vi "Intake Controller.vi"(8 "error in":errorcluster) -> ()   [LabVIEW 2015]
doc: "This VI executes continuously carrying out the current operation and responding to updates or new operations. It will often contain the timing or control code that is difficult to place directly in TeleOp. This VI generally opens all sensors and motors and isolates the rest of the robot code from knowing how the operations are carried out."
uses:
  Intake Setpoints.ctl
  Intake Operations.ctl
  <vilib>/Rock Robotics/WPI/CAN/TalonSRX/WPI_CANTalonSRX_APIControlMode.ctl
  <vilib>/Rock Robotics/WPI/SafetyOutput/WPI_SafetyOutputConfigMenu.ctl
  <vilib>/Rock Robotics/SystemInterfaces/DIO/FPGA_DIOChannel.ctl
  Support Code/OnButton/OnButtonSingle.vi
  Intake Published Globals.vi
  <vilib>/Rock Robotics/WPI/MotorControl/WPI_MotorControlOpenCANTalonSRX.vi
  <vilib>/Rock Robotics/Network Tables/NT Write Boolean.vi
panel:
  out "Current\nCmd":string
  # "Tip: It may be helpful to observe inputs and sensor values.\nYou may also want to display tuning or debugging controls."
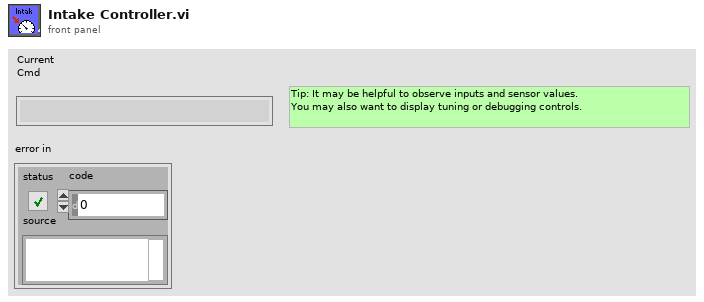
[diagram p1: front panel]
types:
  T1 = typedef "Intake Setpoints.ctl" = cluster{"Operation":T2, "Setpoint":dbl, "Duration":dbl}
  T2 = typedef "Intake Operations.ctl" = enum16{"Reserve", "Read Current", "Immediate", "Idle", "Eject", "Intake", "Queue to Shooter", "Load to Shooter"}
  T3 = typedef "FPGA_DIOChannel.ctl" = enum8{"DIO 0", "DIO 1", "DIO 2", "DIO 3", "DIO 4", "DIO 5", "DIO 6", "DIO 7", "DIO 8", "DIO 9", "DIO MXP 0", "DIO MXP 1", "DIO MXP 2", "DIO MXP 3", "DIO MXP 4", "DIO MXP 5", "DIO MXP 6", "DIO MXP 7", "DIO MXP 8", "DIO MXP 9", "DIO MXP 10", "DIO MXP 11", "DIO MXP 12", "DIO MXP 13", "DIO MXP 14", "DIO MXP 15", "Invalid"}
  T4 = typedef "WPI_SafetyOutputConfigMenu.ctl" = enum16{"Enable", "Disable"}
  T5 = typedef "WPI_CANTalonSRX_APIControlMode.ctl" = enum8{"Percent VBus", "Speed", "Position", "Slave", "Unchanged / Invalid", "Voltage Compensation", "Current", "Motion Profile"}
  T6 = typedef "WPI_DigitalInputDevRef.ctl" = cluster{"DevStatus":errorcluster, "DIO Channel":T3}
  T7 = typedef "WPI_MotorControlDeviceRef.ctl" = cluster{"DeviceStatus":errorcluster, "Type":T8, "PWM":cluster{"PWM Channel":T9, "DeadBand":T10}, "CAN":cluster{"Device Number":u8, "Control Mode":T11, "Semaphore":T12, "Max Vout":dbl, "TalonSRX Control Mode":T5}, "Invert":bool}
  T8 = typedef "WPI_MotorControlType.ctl" = enum16{"PWM", "CAN", "CANTalonSRX"}
  T9 = typedef "FPGA_DIOPWMChannel.ctl" = enum8{"PWM 0", "PWM 1", "PWM 2", "PWM 3", "PWM 4", "PWM 5", "PWM 6", "PWM 7", "PWM 8", "PWM 9", "PWM MXP 0", "PWM MXP 1", "PWM MXP 2", "PWM MXP 3", "PWM MXP 4", "PWM MXP 5", "PWM MXP 6", "PWM MXP 7", "PWM MXP 8", "PWM MXP 9", "Invalid"}
  T10 = typedef "WPI_PWMDeadband.ctl" = cluster{"Name":string, "maxPositivePwm":i32, "minPositivePwm":i32, "centerPwm":i32, "maxNegativePwm":i32, "minNegativePwm":i32, "angularRange":u16}
  T11 = typedef "WPI_CANJaguar_ControlMode.ctl" = enum8{"Percent VBus", "Current", "Speed", "Position", "Voltage"}
  T12 = typedef "Semaphore RefNum" = refnum<k1>
  T13 = typedef "Command Status Info.ctl" = cluster{"Name":string, "Status":T14, "notifier out":T15}
  T14 = typedef "Completion Status.ctl" = enum16{"Successful", "Aborted", "Incomplete"}
  T15 = typedef "Completion Notifier.ctl" = refnum<notifier>
  T16 = cluster{"Default Command":T1, "Command Timing":cluster{"Start Time (ms)":u32, "Iterations":i32}, "Command Arguments":cluster{"Command Info":T13, "Description":string, "Default Command":T1, "notifier out":refnum<notifier>, "Subsystem Name":string}}
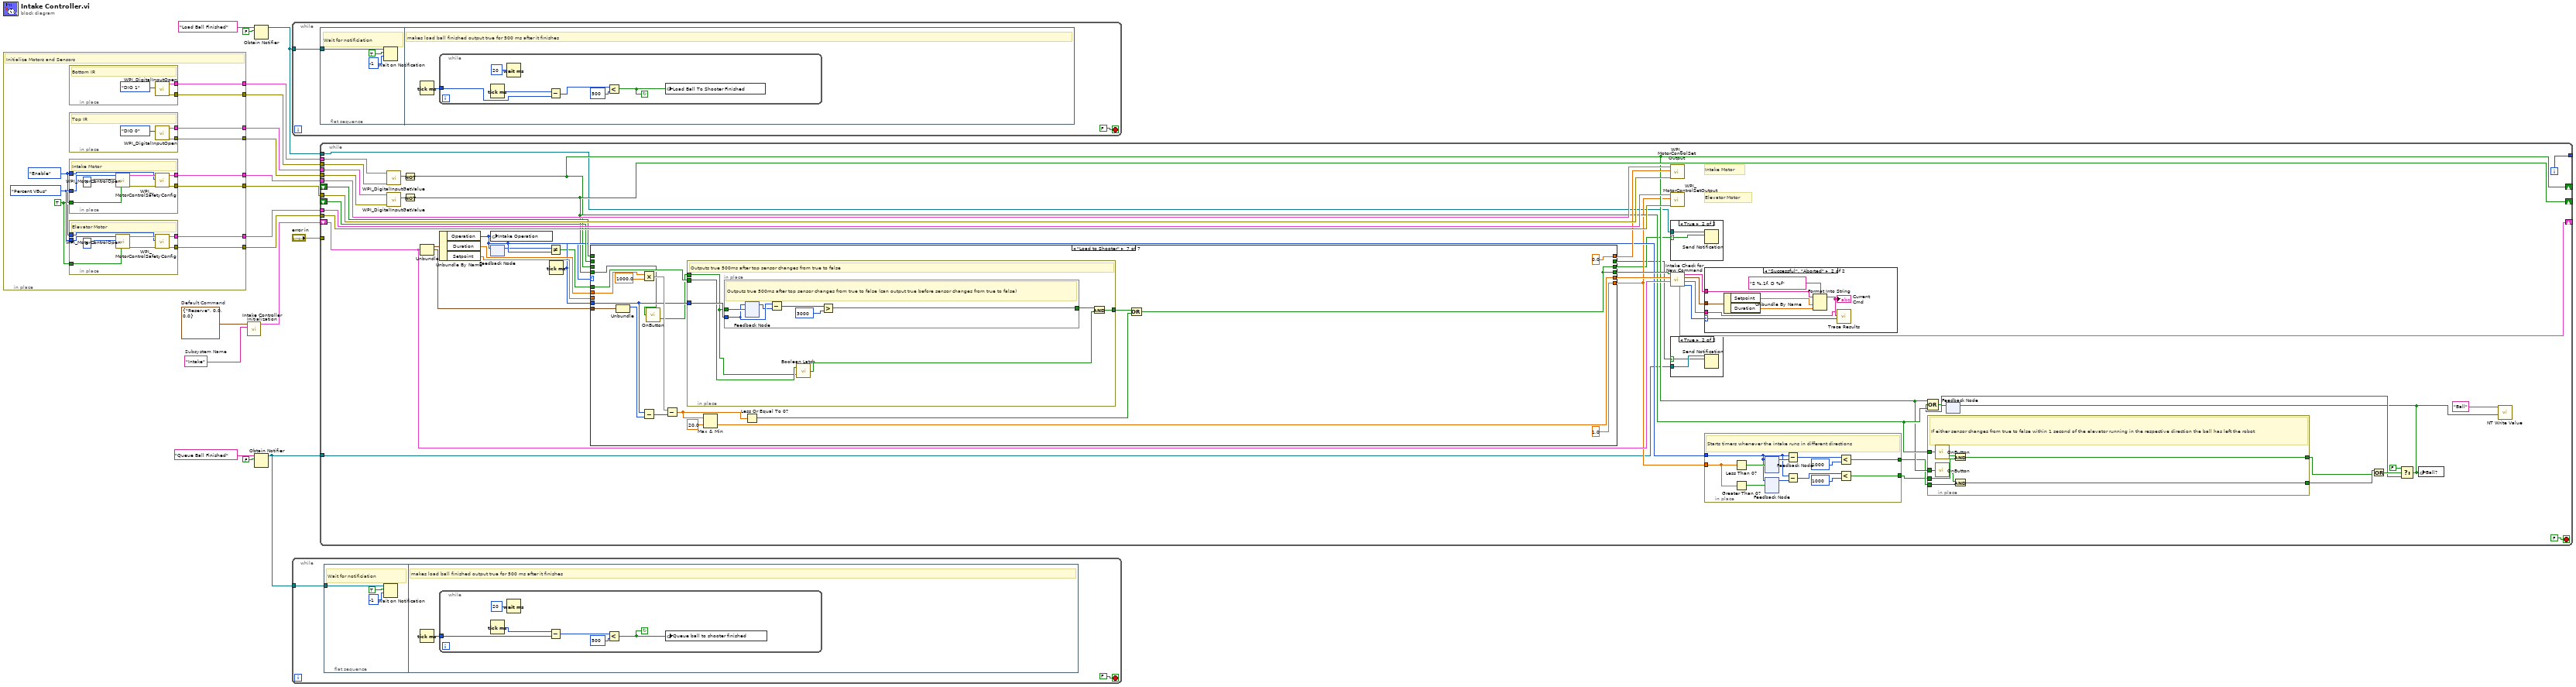
[diagram p0: block diagram]
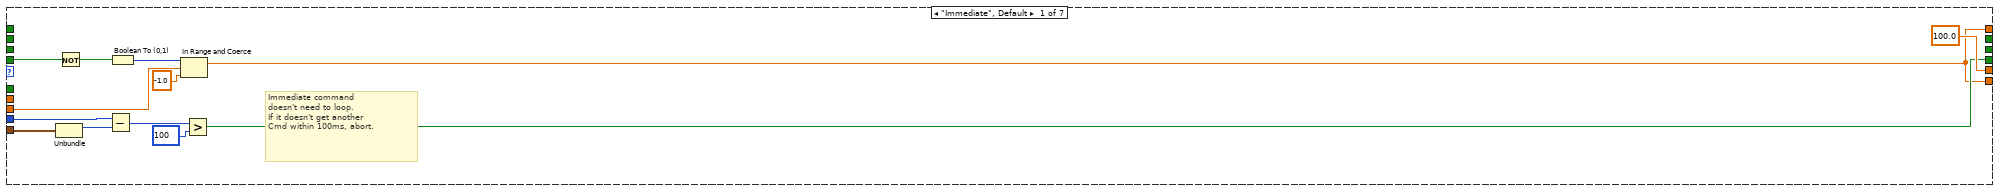
[diagram p5: hidden frame]
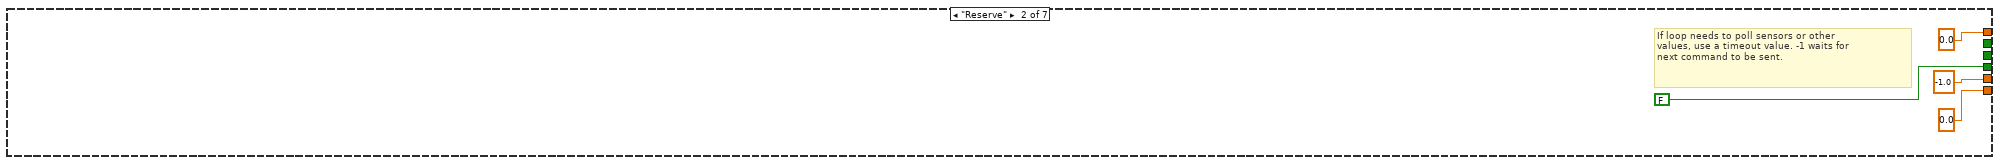
[diagram p6: hidden frame]
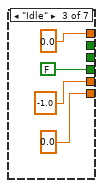
[diagram p7: hidden frame]
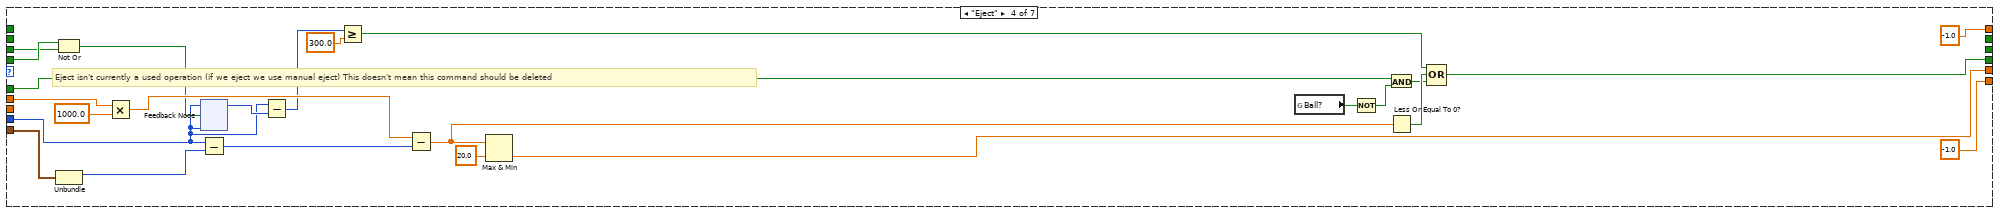
[diagram p8: hidden frame]
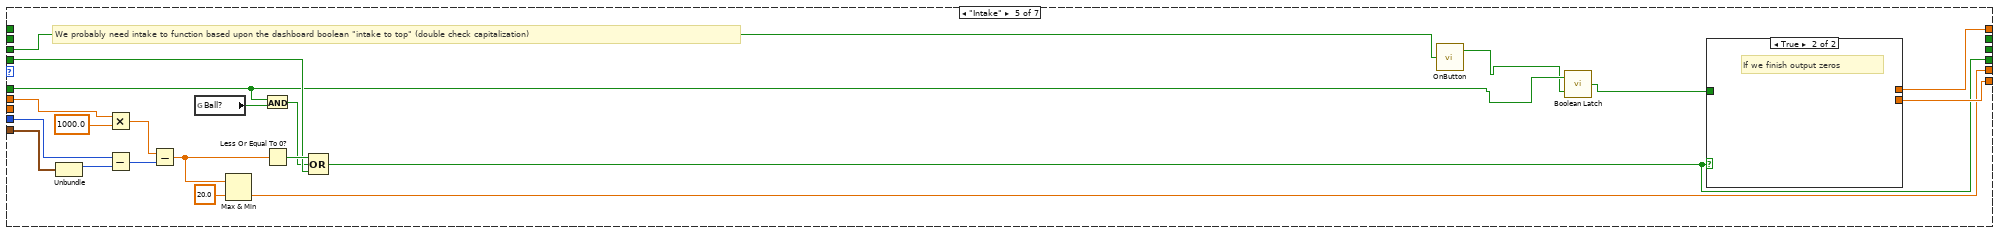
[diagram p9: hidden frame]
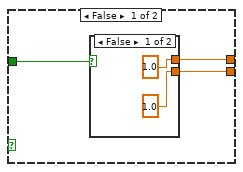
[diagram p10: hidden frame]
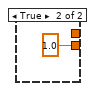
[diagram p11: hidden frame]
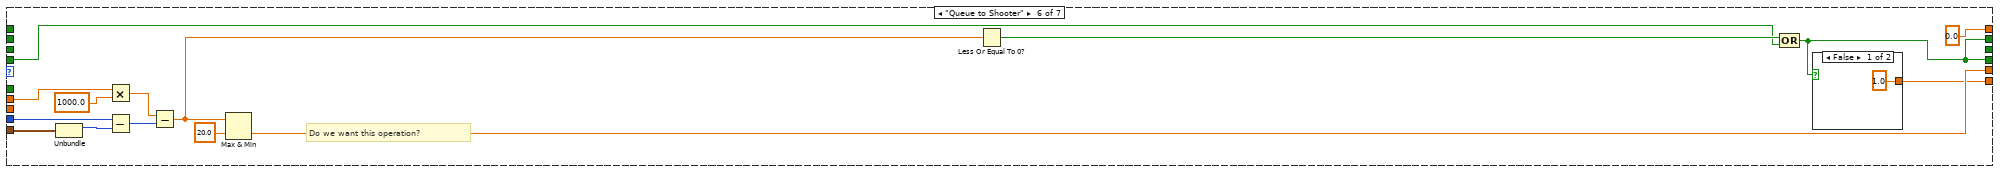
[diagram p12: hidden frame]
diagram:
  w15 = T1 {"Operation"=enum."Reserve", "Setpoint"=0.0, "Duration"=0.0}  # Default Command
  w16 = "Intake"  # Subsystem Name
  n1 = in-place {
    in-place-border: [w29] -> w14
    in-place-border: [w26] -> w13
    in-place-border: [w25] -> w12
    in-place-border: [w24] -> w11
    in-place-border: [w23] -> w10
    in-place-border: [w21] -> w9
    in-place-border: [w20] -> w8
    in-place-border: [w19] -> w7
    w22 = WPI_SafetyOutputConfigMenu."Enable" ("mode")
    w27 = TRUE ("Invert")
    w28 = WPI_CANTalonSRX_APIControlMode."Percent VBus" ("Control Mode")
    # "Initialize Motors and Sensors"
    n2 = in-place {
      in-place-border: [w35] -> w29
      in-place-border: [w34] -> w21
      # "Bottom IR"
      n3 = call <vilib>:"WPI_DigitalInputOpen.vi"("DIO Channel"=FPGA_DIOChannel."DIO 1") -> ("error out"=w34:errorcluster, "DigitalInputDevRef"=w35:T6)  [unwired: 9 in]
    }
    n4 = in-place {
      in-place-border: [w32] -> w20
      in-place-border: [w31] -> w19
      # "Top IR"
      n5 = call <vilib>:"WPI_DigitalInputOpen.vi"("DIO Channel"=FPGA_DIOChannel."DIO 0") -> ("error out"=w32:errorcluster, "DigitalInputDevRef"=w31:T6)  [unwired: 9 in]
    }
    n6 = in-place {
      in-place-border: w28 -> [w51]
      in-place-border: w27 -> [w50]
      in-place-border: [w48] -> w24
      in-place-border: [w46] -> w23
      in-place-border: w22 -> [w45]
      # "Intake Motor"
      n7 = call-poly <vilib>:"WPI_MotorControlOpen.vi"("Invert"=w50, "Device Number"=u8 7, "Control Mode"=w51) -> ("error out"=w49:errorcluster, "MotorControlDeviceRef"=w47:T7)  [unwired: 7 in]
      n8 = call <vilib>:"WPI_MotorControlSafetyConfig.vi"("error in (no error)"=w49, "mode"=w45, "MotorControlDevRef"=w47) -> ("error out"=w48:errorcluster, "MotorControlDevRef"=w46:T7)  [unwired: 7 in]
    }
    n9 = in-place {
      in-place-border: w28 -> [w43]
      in-place-border: w27 -> [w42]
      in-place-border: [w40] -> w26
      in-place-border: [w38] -> w25
      in-place-border: w22 -> [w37]
      # "Elevator Motor"
      n10 = call-poly <vilib>:"WPI_MotorControlOpen.vi"("Invert"=w42, "Device Number"=u8 8, "Control Mode"=w43) -> ("error out"=w39:errorcluster, "MotorControlDeviceRef"=w41:T7)  [unwired: 7 in]
      n11 = call <vilib>:"WPI_MotorControlSafetyConfig.vi"("error in (no error)"=w39, "mode"=w37, "MotorControlDevRef"=w41) -> ("error out"=w38:errorcluster, "MotorControlDevRef"=w40:T7)  [unwired: 7 in]
    }
  }
  n12 = call "Intake Controller Initialization.vi"("Subsystem Name"=w16, "Default Command"=w15) -> ("Command Info"=w17:T16)  [unwired: 9 in]
  n13 = Obtain Notifier(name (unnamed)="Load Ball Finished", notification data type=FALSE) -> (notifier out=w4:refnum<notifier>)  [unwired: 2 in, 2 out]
  n14 = Obtain Notifier(name (unnamed)="Queue Ball Finished", notification data type=FALSE) -> (notifier out=w1:refnum<notifier>)  [unwired: 2 in, 2 out]
  n15 = while {
    tunnel: w4 -> [w53]
    stop <- FALSE stop-if-true
    n16 = flat-sequence {
      tunnel: w53 -> [w56]
      frame #0 {
        # "Wait for notificiation"
        n17 = Wait on Notification(notifier=w56, ignore previous (F)=TRUE, timeout in ms (-1)=-1) -> ()  [unwired: 1 in, 4 out]
      }
      frame #1 {
        # "makes load ball finished output true for 500 ms after it finishes"
        n18 = Tick Count (ms)() -> (millisecond timer value=w57:u32)
        n19 = while {
          tunnel: w57 -> [w59]
          stop <- w63 continue-if-true
          n20 = Tick Count (ms)() -> (millisecond timer value=w58:u32)
          n21 = Wait (ms)(milliseconds to wait=20) -> ()  [unwired: 1 out]
          n22 = Subtract(x=w58, y=w59) -> (x-y=w61:u32)
          n23 = Less?(x=w61, y=u32 500) -> (x < y?=w63:bool)
          n24 = global write "Intake Published Globals.vi" "Load Ball To Shooter Finished"(w63) -> ()
        }
      }
    }
  }
  n25 = while {
    tunnel: w1 -> [w65]
    stop <- FALSE stop-if-true
    n26 = flat-sequence {
      tunnel: w65 -> [w68]
      frame #0 {
        # "Wait for notificiation"
        n27 = Wait on Notification(notifier=w68, ignore previous (F)=TRUE, timeout in ms (-1)=-1) -> ()  [unwired: 1 in, 4 out]
      }
      frame #1 {
        # "makes load ball finished output true for 500 ms after it finishes"
        n28 = Tick Count (ms)() -> (millisecond timer value=w69:u32)
        n29 = while {
          tunnel: w69 -> [w71]
          stop <- w75 continue-if-true
          n30 = Tick Count (ms)() -> (millisecond timer value=w70:u32)
          n31 = Wait (ms)(milliseconds to wait=20) -> ()  [unwired: 1 out]
          n32 = Subtract(x=w70, y=w71) -> (x-y=w73:u32)
          n33 = Less?(x=w73, y=u32 500) -> (x < y?=w75:bool)
          n34 = global write "Intake Published Globals.vi" "Queue ball to shooter finished"(w75) -> ()
        }
      }
    }
  }
  n35 = while {
    shift-right: [w116] -> _
    shift-left: w17 -> [w117]
    tunnel: [w122] -> _
    tunnel: "error in" -> [_]
    tunnel: w14 -> [w109]
    tunnel: w10 -> [w108]
    tunnel: w13 -> [w107]
    tunnel: w12 -> [w106]
    tunnel: w11 -> [w105]
    tunnel: w9 -> [w104]
    tunnel: w8 -> [w103]
    tunnel: w7 -> [w102]
    shift-right: [w95] -> _
    shift-left: _ -> [w99]
    shift-right: [w94] -> _
    shift-left: _ -> [w100]
    tunnel: w4 -> [w92]
    tunnel: w1 -> [w89]
    i -> [w122]
    stop <- FALSE stop-if-true
    # "Intake Motor"
    # "Elevator Motor"
    n36 = call <vilib>:"WPI_DigitalInputGetValue.vi"("error in (no error)"=w104, "DigitalInputDevRef"=w109) -> ("Value"=w76:bool)  [unwired: 7 in, 2 out]
    n37 = call <vilib>:"WPI_DigitalInputGetValue.vi"("error in (no error)"=w103, "DigitalInputDevRef"=w102) -> ("Value"=w77:bool)  [unwired: 7 in, 2 out]
    n38 = Not(x=w76) -> (.not. x?=w94:bool)
    n39 = Not(x=w77) -> (.not. x?=w95:bool)
    n40 = Unbundle(w117) -> ("Default Command"=w121:T1, "Command Timing"=w119:cluster{"Start Time (ms)":u32, "Iterations":i32})  [unwired: 1 out]
    n41 = Unbundle By Name(w121) -> ("Operation"=w90:T2, "Duration"=w120:dbl, "Setpoint"=w118:dbl)
    n42 = global write "Intake Published Globals.vi" "Intake Operation"(w90) -> ()
    n43 = feedback-in #1(w90) -> ()
    n44 = feedback #1() -> (w97:T2)  [unwired: 1 in]
    n45 = Not Equal?(x=w90, y=w97) -> (x != y?=w96:bool)
    n46 = Tick Count (ms)() -> (millisecond timer value=w98:u32)
    n47 = case shown="\"Load to Shooter\"" w90 {
      tunnel: [100.0 -1.0 -1.0 w197 w218 w235 w255] -> w114
      tunnel: [w162 FALSE ("ignore previous (F)") FALSE ("ignore previous (F)") w186 w208 w229 w247] -> w115
      tunnel: w119 -> [w164 _ _ w196 w220 w236 w257]
      tunnel: w120 -> [_ _ _ w195 w219 w238 w256]
      tunnel: w98 -> [w163 _ _ w181 w210 w237 w251]
      tunnel: w118 -> [w157 _ _ _ _ _ _]
      tunnel: w94 -> [_ _ _ w184 w205 _ _]
      tunnel: [w156 0.0 0.0 -1.0 w222 0.0 0.0] -> w101
      tunnel: [w156 0.0 0.0 ("Output") -1.0 ("Output") w221 w233 1.0 ("Output")] -> w93
      tunnel: w95 -> [w160 _ _ w192 w209 w230 w246]
      tunnel: w100 -> [_ _ _ _ _ _ _]
      tunnel: w99 -> [_ _ _ _ _ _ _]
      tunnel: w96 -> [_ _ _ w178 w204 _ w250]
      tunnel: [_ _ _ _ _ _ w247] -> w91
      tunnel: [_ _ _ _ _ w229 _] -> w88
      frame "Immediate", Default {
        # "Immediate command\ndoesn't need to loop.\nIf it doesn't get another\nCmd within 100ms, abort."
        n48 = Unbundle(w164) -> ("Start Time (ms)"=w167:u32)  [unwired: 1 out]
        n49 = Not(x=w160) -> (.not. x?=w159:bool)
        n50 = Subtract(x=w163, y=w167) -> (x-y=w166:u32)
        n51 = Boolean To (0,1)(Boolean=w159) -> (0, 1=w158:i16)
        n52 = In Range and Coerce(upper limit=w158, x=w157, lower limit=-1.0) -> (coerced(x)=w156:dbl)  [unwired: 1 out]
        n53 = Greater?(x=w166, y=u8 100 ("Left Motor")) -> (0:w162:bool)
      }
      frame "Reserve" {
        # "If loop needs to poll sensors or other\nvalues, use a timeout value. -1 waits for\nnext command to be sent."
      }
      frame "Idle" {
      }
      frame "Eject" {
        # "Eject isn't currently a used operation (if we eject we use manual eject) This doesn't mean this command should be deleted"
        n54 = Not Or(1:w184, 2:w192) -> (0:w183:bool)
        n55 = Unbundle(w196) -> ("Start Time (ms)"=w199:u32)  [unwired: 1 out]
        n56 = Multiply(x=w195, y=1000.0) -> (x*y=w191:dbl)
        n57 = feedback-in #2(w181, w183) -> ()
        n58 = feedback #2(w181) -> (w182:u32)
        n59 = Subtract(x=w181, y=w199) -> (x-y=w201:u32)
        n60 = Subtract(x=w181, y=w182) -> (x-y=w189:u32)
        n61 = Greater Or Equal?(x=w189, y=300.0) -> (x >= y?=w185:bool)
        n62 = Subtract(x=w191, y=w201) -> (x-y=w188:dbl)
        n63 = Max & Min(x=w188, y=20.0) -> (min(x,y)=w197:dbl)  [unwired: 1 out]
        n64 = global read "Intake Published Globals.vi" "Ball?"() -> (w180:bool)
        n65 = Not(x=w180) -> (.not. x?=w179:bool)
        n66 = And(x=w178, y=w179) -> (x .and. y?=w177:bool)
        n67 = Less Or Equal To 0?(x=w188) -> (x <= 0?=w187:bool)
        n68 = Compound Arithmetic op=OR(w185, w187, w177) -> (w186:bool)
      }
      frame "Intake" {
        # "We probably need intake to function based upon the dashboard boolean \"intake to top\" (double check capitalization)"
        n69 = Unbundle(w220) -> ("Start Time (ms)"=w214:u32)  [unwired: 1 out]
        n70 = Multiply(x=w219, y=1000.0) -> (x*y=w216:dbl)
        n71 = Subtract(x=w210, y=w214) -> (x-y=w217:u32)
        n72 = Subtract(x=w216, y=w217) -> (x-y=w211:dbl)
        n73 = global read "Intake Published Globals.vi" "Ball?"() -> (w207:bool)
        n74 = Max & Min(x=w211, y=20.0) -> (min(x,y)=w218:dbl)  [unwired: 1 out]
        n75 = And(x=w204, y=w207) -> (x .and. y?=w206:bool)
        n76 = Less Or Equal To 0?(x=w211) -> (x <= 0?=w212:bool)
        n77 = Compound Arithmetic op=OR(w212, w206, w209) -> (w208:bool)
        n78 = call-poly "OnButton.vi"("Input"=w205) -> ("Pressed"=w203:bool)  [unwired: 1 out]
        n79 = call "Boolean Latch.vi"("Input"=w203, "Reset"=w204) -> ("Output"=w202:bool)
        n80 = case shown="True" w208 {
          tunnel: [w225 _] -> w222
          tunnel: [w224 _] -> w221
          tunnel: w202 -> [w223 _]
          frame False {
            n81 = case shown="False" w223 {
              tunnel: [1.0 _] -> w225
              tunnel: [1.0 ("Output") 1.0] -> w224
              frame False {
              }
              frame True {
              }
            }
          }
          frame True {
            # "If we finish output zeros"
          }
        }
      }
      frame "Queue to Shooter" {
        # "Do we want this operation?"
        n82 = Unbundle(w236) -> ("Start Time (ms)"=w240:u32)  [unwired: 1 out]
        n83 = Multiply(x=w238, y=1000.0) -> (x*y=w242:dbl)
        n84 = Subtract(x=w237, y=w240) -> (x-y=w243:u32)
        n85 = Subtract(x=w242, y=w243) -> (x-y=w232:dbl)
        n86 = Max & Min(x=w232, y=20.0) -> (min(x,y)=w235:dbl)  [unwired: 1 out]
        n87 = Less Or Equal To 0?(x=w232) -> (x <= 0?=w231:bool)
        n88 = Compound Arithmetic op=OR(w231, w230) -> (w229:bool)
        n89 = case shown="False" w229 {
          tunnel: [1.0 _] -> w233
          frame False {
          }
          frame True {
          }
        }
      }
      frame "Load to Shooter" {
        n90 = Unbundle(w257) -> ("Start Time (ms)"=w259:u32)  [unwired: 1 out]
        n91 = Multiply(x=w256, y=1000.0) -> (x*y=w261:dbl)
        n92 = Subtract(x=w251, y=w259) -> (x-y=w262:u32)
        n93 = call-poly "OnButton.vi"("Input"=w246) -> ("Released"=w245:bool)  [unwired: 1 out]
        n94 = Subtract(x=w261, y=w262) -> (x-y=w252:dbl)
        n95 = in-place {
          in-place-border: w250 -> [w265]
          in-place-border: w251 -> [w268]
          in-place-border: [w267] -> w249
          in-place-border: w245 -> [w264]
          # "Outputs true 500ms after top sensor changes from true to false"
          n96 = in-place {
            in-place-border: w264 -> [w274]
            in-place-border: w268 -> [w273]
            in-place-border: [w269] -> w266
            # "Outputs true 500ms after top sensor changes from true to false (can output true before sensor changes from true to false)"
            n97 = feedback #3() -> (w272:u32)  [unwired: 1 in]
            n98 = feedback-in #3(w273, w274) -> ()
            n99 = Subtract(x=w273, y=w272) -> (x-y=w271:u32)
            n100 = Greater?(x=w271, y=u32 3000) -> (0:w269:bool)
          }
          n101 = call "Boolean Latch.vi"("Input"=w264, "Reset"=w265) -> ("Output"=w263:bool)
          n102 = And(x=w266, y=w263) -> (x .and. y?=w267:bool)
        }
        n103 = Max & Min(x=w252, y=20.0) -> (min(x,y)=w255:dbl)  [unwired: 1 out]
        n104 = Less Or Equal To 0?(x=w252) -> (x <= 0?=w248:bool)
        n105 = Compound Arithmetic op=OR(w249, w248) -> (w247:bool)
      }
    }
    n106 = call <vilib>:"WPI_MotorControlSetOutput.vi"("error in (no error)"=w105, "Output"=w101, "MotorControlDevRef"=w108) -> ()  [unwired: 6 in, 3 out]
    n107 = call <vilib>:"WPI_MotorControlSetOutput.vi"("error in (no error)"=w106, "Output"=w93, "MotorControlDevRef"=w107) -> ()  [unwired: 6 in, 3 out]
    n108 = case shown="True" w91 {
      selector: w91 -> [_ w146]
      tunnel: w92 -> [_ w147]
      frame False {
      }
      frame True {
        n109 = Send Notification(notification=w146, notifier=w147) -> ()  [unwired: 1 in, 2 out]
      }
    }
    n110 = call "Intake Check for New Command.vi"("Current Command"=w117, "Wait time (ms)"=w114, "Finished?"=w115) -> ("Completion"=w110:T14, "Subsystem Name"=w111:string, "Current Command"=w112:T1, "Initial Trace String"=w113:string, "NextCommand"=w116:T16)  [unwired: 4 in]
    n111 = case shown="True" w88 {
      selector: w88 -> [_ w144]
      tunnel: w89 -> [_ w145]
      frame False {
      }
      frame True {
        n112 = Send Notification(notification=w144, notifier=w145) -> ()  [unwired: 1 in, 2 out]
      }
    }
    n113 = case shown="\"Successful\", \"Aborted\"" w110 {
      selector: w110 -> [_ w155]
      tunnel: w113 -> [_ w151]
      tunnel: w112 -> [_ w152]
      tunnel: w111 -> [_ w148]
      frame "Incomplete", Default {
        # "Continuing current command"
      }
      frame "Successful", "Aborted" {
        # "Report and setup for next command"
        n114 = Unbundle By Name(w152) -> ("Setpoint"=w154:dbl, "Duration"=w149:dbl)
        n115 = Format Into String(format string="S %.1f, D %f", initial string=w151, w154, w149) -> (resulting string=w150:string)  [unwired: 1 in, 1 out]
        "Current\nCmd" <- w150
        n116 = call <vilib>:"Trace Results.vi"("Status of previous command"=w155, "Description"=w150, "Subsystem"=w148) -> ()  [unwired: 9 in]
      }
    }
    n117 = in-place {
      in-place-border: w93 -> [w143]
      in-place-border: w98 -> [w132]
      in-place-border: [w136] -> w87
      in-place-border: [w133] -> w86
      # "Starts timers whenever the intake runs in different directions"
      n118 = Less Than 0?(x=w143) -> (x < 0?=w135:bool)
      n119 = Greater Than 0?(x=w143) -> (x > 0?=w134:bool)
      n120 = feedback #4() -> (w142:u32)  [unwired: 1 in]
      n121 = feedback-in #4(w132, w135) -> ()
      n122 = feedback #5() -> (w138:u32)  [unwired: 1 in]
      n123 = feedback-in #5(w132, w134) -> ()
      n124 = Subtract(x=w132, y=w142) -> (x-y=w141:u32)
      n125 = Subtract(x=w132, y=w138) -> (x-y=w137:u32)
      n126 = Less?(x=w141, y=u32 1000) -> (x < y?=w136:bool)
      n127 = Less?(x=w137, y=u32 1000) -> (x < y?=w133:bool)
    }
    n128 = in-place {
      in-place-border: w87 -> [w131]
      in-place-border: w95 -> [w126]
      in-place-border: w86 -> [w130]
      in-place-border: [w129] -> w85
      in-place-border: [w128] -> w84
      in-place-border: w94 -> [w127]
      # "If either sensor changes from true to false within 1 second of the elevator running in the respective direction the ball has left the robot"
      n129 = call-poly "OnButton.vi"("Input"=w126) -> ("Released"=w124:bool)  [unwired: 1 out]
      n130 = call-poly "OnButton.vi"("Input"=w127) -> ("Released"=w125:bool)  [unwired: 1 out]
      n131 = And(x=w124, y=w130) -> (x .and. y?=w128:bool)
      n132 = And(x=w125, y=w131) -> (x .and. y?=w129:bool)
    }
    n133 = feedback #6() -> (w81:bool)  [unwired: 1 in]
    n134 = Compound Arithmetic op=OR(w94, w81, w95) -> (w80:bool)
    n135 = Or(x=w85, y=w84) -> (x .or. y?=w83:bool)
    n136 = Select(t=FALSE, s=w83, f=w80) -> (s? t:f=w78:bool)
    n137 = feedback-in #6(w78) -> ()
    n138 = global write "Intake Published Globals.vi" "Ball?"(w78) -> ()
    n139 = call-poly <vilib>:"NT Write Value.vi"("Boolean"=w78, "Name"="Ball") -> ()  [unwired: 9 in, 1 out]
  }
